vi "createResponseParser.vi"(8 "error in (no error)":errorcluster, 11 "ModernOvenFactory In":refnum<class "ModernOvenFactory.lvclass">) -> (0 "error out":errorcluster, 2 "responseParser":refnum<class "IResponseParser.lvclass">, 3 "ModernOvenFactory Out":refnum<class "ModernOvenFactory.lvclass">)   [LabVIEW 2023, in "AbstractFactory.lvlib" / "ModernOvenFactory.lvclass"]
uses:
  ModernOvenFactory.lvclass
  IResponseParser/IResponseParser.lvclass
  ModernOvenFactory.lvclass/ModernOvenFactory.ctl
  XMLResponseParser/XMLResponseParser.lvclass
  C:/projects/DesignPatterns_LabVIEW/AbstractFactory/XMLResponseParser/XMLResponseParser.lvclass
  C:/projects/DesignPatterns_LabVIEW/AbstractFactory/IResponseParser/IResponseParser.lvclass
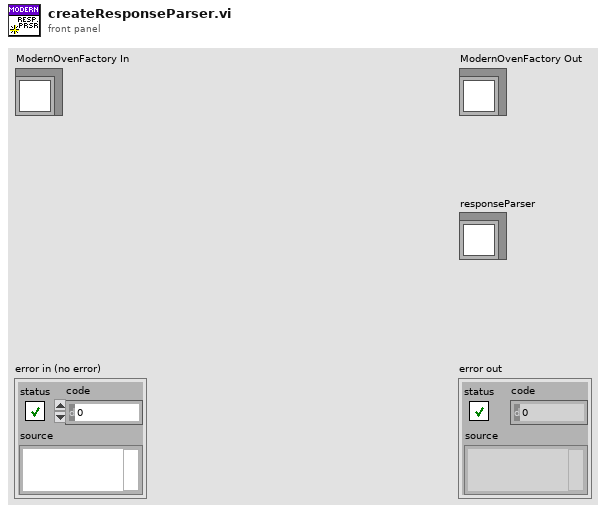
[diagram p1: front panel]
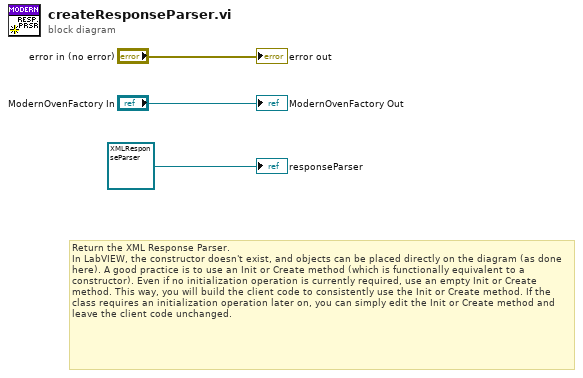
[diagram p0: block diagram]
diagram:
  # "Return the XML Response Parser.\nIn LabVIEW, the constructor doesn't exist, and objects can be placed directly on the diagram (as done here). A good practice is to use an Init or Create method (which is functionally equivalent to a constructor). Even if no initialization operation is currently required, use an empty Init or Create method. This way, you will build the client code to consistently use the Init or Create method. If the class requires an initialization operation later on, you can simply edit the Init or Create method and leave the client code unchanged."
  "error out" <- "error in (no error)"
  "ModernOvenFactory Out" <- "ModernOvenFactory In"
  "responseParser" <- refnum<class "XMLResponseParser.lvclass"> refnum ("AbstractFactory.lvlib:XMLResponseParser.lvclass")
